vi "Network Engine.vi"(10 "Parameters":variant, 11 "Process":refnum<class "Process.lvclass">) -> ()   [LabVIEW 2019, in "Control Addon Engine.lvlib"]
uses:
  Control Addon Engine.lvlib
  <vilib>/NI/NIVS Inline Async API/_VS Inline Async API/Process/Process.lvclass
  Types/RT Configuration.ctl
  Addon Shared/Types/Gain Schedule.ctl
  Addon Shared/Types/Compiled Settings.ctl
  Addon Shared/Types/Compiled PID Settings.ctl
  <vilib>/NI VeriStand/Custom Device API/Block Data Reference.ctl
  <vilib>/NI VeriStand/Custom Device API/Data Reference.ctl
  Addon Shared/Types/Compiled Industrial Settings.ctl
  Addon Shared/Types/Compiled Industrial Parameters.ctl
  <vilib>/NI/NI VeriStand Addon Network Comm/Engine/VeriStand Comm.lvclass/VeriStand Comm.ctl
  <vilib>/NI/NIVS Inline Async API/_VS Inline Async API/Process/Process.lvclass/Process.ctl
  Format Debug String.vi
  <vilib>/NI/NIVS Inline Async API/_VS Inline Async API/Process/Methods/Async.Processes.WaitonStart.vi
  <vilib>/NI/NI VeriStand Addon Network Comm/Engine/Process/Initialize Comm Refs.vi
  <vilib>/NI/NI VeriStand Addon Network Comm/Engine/_SubVIs/Comm Connection Engine.vi
  <vilib>/NI/NI VeriStand Addon Network Comm/Engine/_SubVIs/Comm Command Engine.vi
  <vilib>/NI/NIVS Inline Async API/_VS Inline Async API/Error Handling Process/SubVIs/Error.ConvertArray.vi
  <vilib>/NI/STM/Connection Manager/TCP/Advanced/TCP Connection Manager (By Reference).vi
  <vilib>/Utility/error.llb/Clear Errors.vi
  <vilib>/NI/STM/Get Connection Reference.vi
  <vilib>/NI/STM/TCP/Get Connection Reference (TCP).vi
  <vilib>/NI/STM/Read Meta Data.vi
  <vilib>/NI/STM/TCP/Read Meta Data (TCP Ref).vi
  <vilib>/NI/NIVS Inline Async API/_VS Inline Async API/Process/Methods/Async.Processes.Report.vi
  <vilib>/NI/AMC/Send Local Message.vi
  <vilib>/NI/Tools/Keyed Array/Add.vi
  <vilib>/NI/AMC/Read Next Message.vi
  <vilib>/NI/STM/Connection Manager/TCP/Advanced/TCP Check Connection (By Reference).vi
  <vilib>/NI/STM/SubVIs/Generate STM Error.vi
  <vilib>/NI/AMC/Create Single Message.vi
  <vilib>/NI/AMC/Update Message Routing Info.vi
  <vilib>/NI/Tools/Keyed Array/Map String.vi
  <vilib>/NI/AMC/Read Termination Message.vi
  <vilib>/NI/Tools/String/Get Case Matching.vi
  <vilib>/Utility/SystemLogging/Write to System Log.vi
  <vilib>/NI/AMC/Create Message Queue.vi
  <vilib>/NI/STM/Connection Manager/TCP/Advanced/TCP Initialize Connection Manager (By Reference).vi
  <vilib>/NI/STM/Read Message.vi
  <vilib>/NI/STM/TCP/Read Message (TCP).vi
  <vilib>/NI/AMC/Send Message.vi
  <vilib>/NI/NI VeriStand Addon Network Comm/Shared/Comm Constants.vi
  <vilib>/NI/AMC/Globals.vi
  <vilib>/NI/STM/Write Message.vi
  <vilib>/NI/STM/TCP/Write Message (TCP).vi
  <vilib>/NI/AMC/Destroy Message Queue.vi
  <vilib>/NI/STM/TCP/Read Meta Data (TCP Clst).vi
  <vilib>/NI/NI VeriStand Addon Network Comm/Engine/Process/Close Comm Refs.vi
  <vilib>/NI/NI VeriStand Addon Network Comm/Engine/VeriStand Comm.lvclass
  Addon Shared/Control Addon Shared.lvlib
  <vilib>/NI VeriStand/Custom Device API/Custom Device API.lvlib
panel:
  out "error out":errorcluster
  in  "error in (no error)":errorcluster
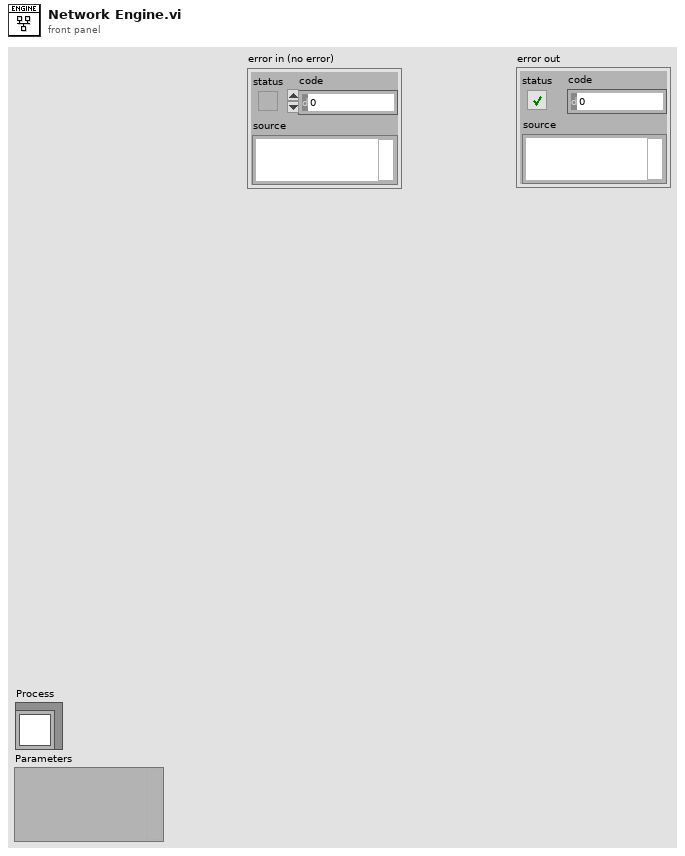
[diagram p1: front panel]
types:
  T1 = typedef "Control Addon Engine.lvlib/RT Configuration.ctl" = cluster{"Parameter Refs":refnum<data-value>[], "Config":T2}
  T2 = typedef "Control Addon Shared.lvlib/Compiled Settings.ctl" = cluster{"PID Settings":T3, "Name":string, "Industrial Settings":T7}
  T3 = typedef "Control Addon Shared.lvlib/Compiled PID Settings.ctl" = cluster{"Gain Schedule":T4[], "Enable Live Updates":bool[], "output range":cluster{"output high":dbl, "output low":dbl}[], "setpoint range":cluster{"setpoint high":dbl, "setpoint low":dbl}[], "Write Refs":T5[], "Write Data":dbl[], "Read Refs":T5[], "Read Data":dbl[], "Control Loop Names":string[], "Enable Gain Scheduling":bool[], "Output Rate Limiter":dbl[], "dt":dbl, "setpoint high limit":dbl[], "setpoint low limit":dbl[], "output high limit":dbl[], "output low limit":dbl[]}
  T4 = typedef "Control Addon Shared.lvlib/Gain Schedule.ctl" = cluster{"Gain Schedule":cluster{"PID gains":cluster{"proportional gain (Kc)":dbl, "integral time (Ti, min)":dbl, "derivative time (Td, min)":dbl}, "max value":dbl}[]}
  T5 = typedef "Custom Device API.lvlib/Block Data Reference.ctl" = cluster{"Data Reference":T6, "Offset":u64, "Length":u64}
  T6 = typedef "Custom Device API.lvlib/Data Reference.ctl" = i32
  T7 = typedef "Control Addon Shared.lvlib/Compiled Industrial Settings.ctl" = cluster{"output range":cluster{"output high":dbl, "output low":dbl}[], "setpoint range":cluster{"setpoint high":dbl, "setpoint low":dbl}[], "Write Refs":T5[], "Write Data":dbl[], "Read Refs":T5[], "Read Data":dbl[], "Control Loop Names":string[], "Parameters":T8[], "Previous States":bool[], "Previous Counts":u64[]}
  T8 = typedef "Control Addon Shared.lvlib/Compiled Industrial Parameters.ctl" = cluster{"Enable Hysteresis":bool, "Hysteresis":dbl, "Minimum Switching":u64}
  T9 = typedef "Control Addon Engine.lvlib/Network Engine State Variables.ctl" = cluster{"Process":refnum<class "Process.lvclass">, "Comm":refnum<class "VeriStand Comm.lvclass">}
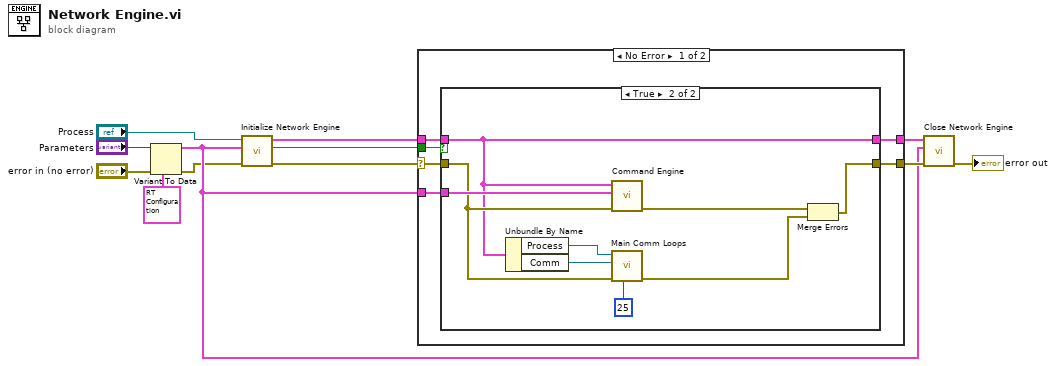
[diagram p0: block diagram]
diagram:
  n1 = Variant To Data(error in="error in (no error)", type=T1 {"Parameter Refs"=[], "Config"={"PID Settings"={"Gain Schedule"=[], "Enable Live Updates"=[], "output range"=[], "setpoint range"=[], "Write Refs"=[], "Write Data"=[], "Read Refs"=[], "Read Data"=[], "Control Loop Names"=[], "Enable Gain Scheduling"=[], "Output Rate Limiter"=[], "dt"=0.0, "setpoint high limit"=[], "setpoint low limit"=[], "output high limit"=[], "output low limit"=[]}, "Name"="", "Industrial Settings"={"output range"=[], "setpoint range"=[], "Write Refs"=[], "Write Data"=[], "Read Refs"=[], "Read Data"=[], "Control Loop Names"=[], "Parameters"=[], "Previous States"=[], "Previous Counts"=[]}}} ("Parameters"), Variant="Parameters") -> (data=w3:T1, error out=w1:errorcluster)
  n2 = call "Initialize Network Engine.vi"("error in (no error)"=w1, "Parameters"=w3, "Process"="Process") -> ("error out"=w8:errorcluster, "Start"=w6:bool, "State Variables"=w12:T9)  [unwired: 6 in]
  n3 = case shown="No Error" w8 {
    selector: w8 -> [w16 w31]
    tunnel: w12 -> [w15 w30]
    tunnel: [w13 w30] -> w11
    tunnel: w3 -> [w18 _]
    tunnel: [w17 w31] -> w9
    tunnel: w6 -> [w14 _]
    frame No Error {
      n4 = case shown="True" w14 {
        tunnel: w18 -> [_ w29]
        tunnel: [w20 w28] -> w17
        tunnel: w16 -> [w20 w26]
        tunnel: w15 -> [w19 w24]
        tunnel: [w19 w24] -> w13
        frame False {
        }
        frame True {
          n5 = Unbundle By Name(w24) -> ("Process"=w23:refnum<class "Process.lvclass">, "Comm"=w21:refnum<class "VeriStand Comm.lvclass">)
          n6 = call "Command Engine.vi"("error in (no error)"=w26, "Parameters"=w29, "State Variables"=w24) -> ("error out"=w27:errorcluster)  [unwired: 8 in]
          n7 = call <vilib>:"Main Comm Loops.vi"("Update Rate"=u32 25, "error in (no error)"=w26, "Comm.lvclass"=w21, "Process"=w23) -> ("error out"=w25:errorcluster)  [unwired: 7 in]
          n8 = Merge Errors(w27, w25) -> (w28:errorcluster)
        }
      }
    }
    frame Error {
    }
  }
  n9 = call "Close Network Engine.vi"("error in (no error)"=w9, "Parameters"=w3, "State Variables"=w11) -> ("error out"=→"error out":errorcluster)  [unwired: 8 in]
